vi "lj_release_resources.vi"(8 "error in (no error)":errorcluster, 11 "LabJackRes":T1) -> (0 "error out":errorcluster)   [LabVIEW 2025, in "LabJackEKG.lvlib"]
uses:
  LabJackEKG.lvlib
  Typedefs/LabJackGlobalResources.ctl
  Typedefs/CounterQueues.ctl
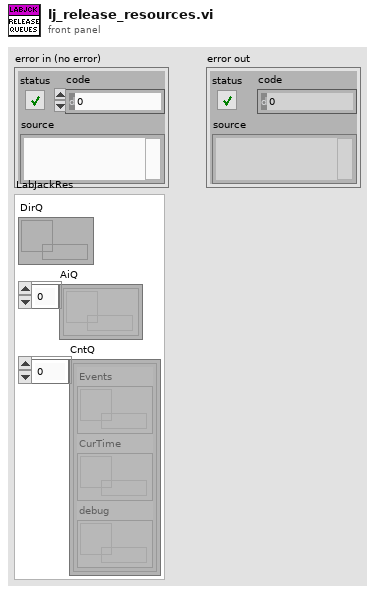
[diagram p1: front panel]
types:
  T1 = typedef "LabJackEKG.lvlib/LabJackGlobalResources.ctl" = cluster{"DirQ":refnum<queue>, "AiQ":refnum<queue>[], "CntQ":T2[]}
  T2 = typedef "LabJackEKG.lvlib/CounterQueues.ctl" = cluster{"Events":refnum<queue>, "CurTime":refnum<queue>, "debug":refnum<queue>}
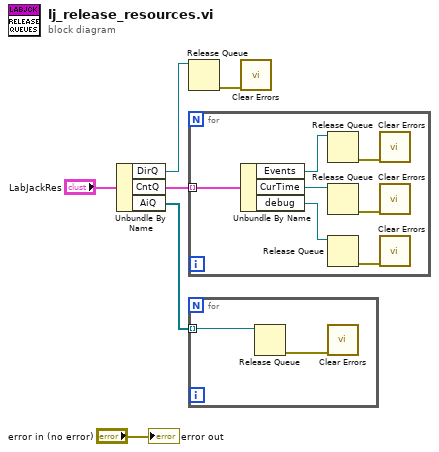
[diagram p0: block diagram]
diagram:
  n1 = Unbundle By Name("LabJackRes") -> ("DirQ"=w5:refnum<queue>, "CntQ"=w4:T2[], "AiQ"=w3:refnum<queue>[])
  n2 = Release Queue(queue=w5) -> (error out=w2:errorcluster)  [unwired: 2 in, 2 out]
  n3 = for {
    tunnel: w4 -> [w12] mode=indexing
    n4 = Unbundle By Name(w12) -> ("Events"=w11:refnum<queue>, "CurTime"=w10:refnum<queue>, "debug"=w7:refnum<queue>)
    n5 = Release Queue(queue=w11) -> (error out=w13:errorcluster)  [unwired: 2 in, 2 out]
    n6 = Release Queue(queue=w10) -> (error out=w9:errorcluster)  [unwired: 2 in, 2 out]
    n7 = Release Queue(queue=w7) -> (error out=w8:errorcluster)  [unwired: 2 in, 2 out]
    n8 = call <vilib>:"Clear Errors.vi"("error in (no error)"=w13) -> ()  [unwired: 5 in, 2 out]
    n9 = call <vilib>:"Clear Errors.vi"("error in (no error)"=w9) -> ()  [unwired: 5 in, 2 out]
    n10 = call <vilib>:"Clear Errors.vi"("error in (no error)"=w8) -> ()  [unwired: 5 in, 2 out]
  }
  n11 = for {
    tunnel: w3 -> [w14] mode=indexing
    n12 = Release Queue(queue=w14) -> (error out=w15:errorcluster)  [unwired: 2 in, 2 out]
    n13 = call <vilib>:"Clear Errors.vi"("error in (no error)"=w15) -> ()  [unwired: 5 in, 2 out]
  }
  n14 = call <vilib>:"Clear Errors.vi"("error in (no error)"=w2) -> ()  [unwired: 5 in, 2 out]
  "error out" <- "error in (no error)"
